vi "Test Copy from Pixmap ARGB.vi"(8 "error in (no error)":errorcluster, 11 "Test Case In":refnum<class "Image.lvclass">) -> (0 "error out":errorcluster, 3 "Test Case Out":refnum<class "Image.lvclass">)   [LabVIEW 2020, in "g_ar_toolkit.test.lvlib" / "Image.lvclass"]
uses:
  Image.lvclass
  C:/Program Files (x86)/National Instruments/LabVIEW 2020/vi.lib/Astemes/LUnit/Test Case.lvclass
  <vilib>/picture/picture.llb/imagedata.ctl
  <vilib>/Astemes/LUnit/Test Case.lvclass/Test Case.ctl
  2c93f62b-78d7-4b59-b27c-14bd701a5d71.vi
  26ba0610-68e5-456e-b31e-3dd4b1a41919.vi
  50a666bd-4679-4783-837b-c667b5268c61.vi
  5112621f-71fb-42da-a54b-011c251ba454.vi
  935961b4-3727-4f5b-bf0e-a61aebcf0dca.vi
  g_ar_toolkit.image/CreateEmptyImageARGB.vi
  g_ar_toolkit.image/CreateEmptyImageGreyscale.vi
  g_ar_toolkit.image/CopyPixmapToImageOuptutMaskARGB.vi
  g_ar_toolkit.image/CopyPixmapToImageFlattenMaskARGB.vi
  7f5bb767-9dbf-47d9-8f44-5f4901e96d00.vi
  e6d5ae8e-bd70-4c65-a769-b7cfb03e80c7.vi
  d454bffa-6717-48ab-b8d5-b1f03345aa55.vi
  g_ar_toolkit.image/CreateEmptyImageARGB.vi/3321fa97-f432-4e1e-8db9-a0df79aed21b.vi
  g_ar_toolkit.image/CreateEmptyImageGreyscale.vi/6598b9e0-8a08-46f5-91fd-ca1b87217137.vi
  g_ar_toolkit.image/CopyPixmapToImageOuptutMaskARGB.vi/80b1166a-8c06-443b-b271-eb6a715622f7.vi
  g_ar_toolkit.image/CopyPixmapToImageFlattenMaskARGB.vi/80b1166a-8c06-443b-b271-eb6a715622f7.vi
  <vilib>/Astemes/LUnit/Append Pass Result.vi
  <vilib>/Astemes/LUnit/Append Fail Result.vi
  <vilib>/Astemes/LUnit/Describe Comparison.vi
  <vilib>/Astemes/LUnit/Compare Variants.vi
  g_ar_toolkit.image/FixPixmap.vi
  <vilib>/Astemes/LUnit/Variant to string.vi
  g_ar_toolkit.image/Default8bitColourMap.vi
  g_ar_toolkit.image/ARGBColourToU32.vi
  <vilib>/Utility/error.llb/Error Cluster From Error Code.vi
  <vilib>/Utility/Data Type/Get Type Information.vi
  <vilib>/Utility/LVClass/Get LV Class Name.vi
  Image.lvclass/Image.ctl
  g_ar_toolkit.image/g_ar_toolkit.image.lvlib
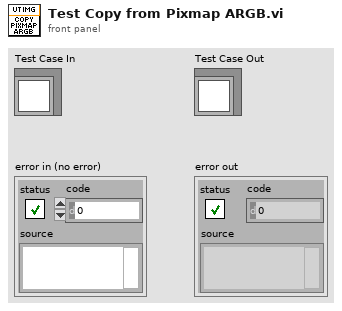
[diagram p1: front panel]
types:
  T1 = enum16{"8 Bit No Mask", "24 Bit No Mask", "32 Bit No Mask", "8 Bit Mask", "24 Bit Mask", "32 Bit Mask", "8 Pixels Wide Masked", "16 Pixels Wide Masked", "8 Bit No Colour Map"}
  T2 = typedef "imagedata.ctl" = cluster{"image type":i32, "image depth":i32, "image":u8[], "mask":u8[], "colors":u32[], "Rectangle":cluster{"left":i16, "top":i16, "right":i16, "bottom":i16}}
  T3 = cluster{"8 No Mask":T2, "8 Mask":T2, "24 No Mask":T2, "24 Mask":T2, "32 No Mask":T2, "32 Mask":T2, "24 Mask - 8 wide":T2, "24 Mask - 16 wide":T2, "8 Bit No Colour Map":T2}
  T4 = cluster{"left":i16, "top":i16, "right":i16, "bottom":i16}
  T5 = enum16{"8 Bit No Mask", "24 Bit No Mask", "32 Bit No Mask", "8 Bit Mask", "24 Bit Mask", "32 Bit Mask", "8 Pixels Wide Masked", "16 Pixels Wide Masked", "8 Bit No Colour Map"}[]
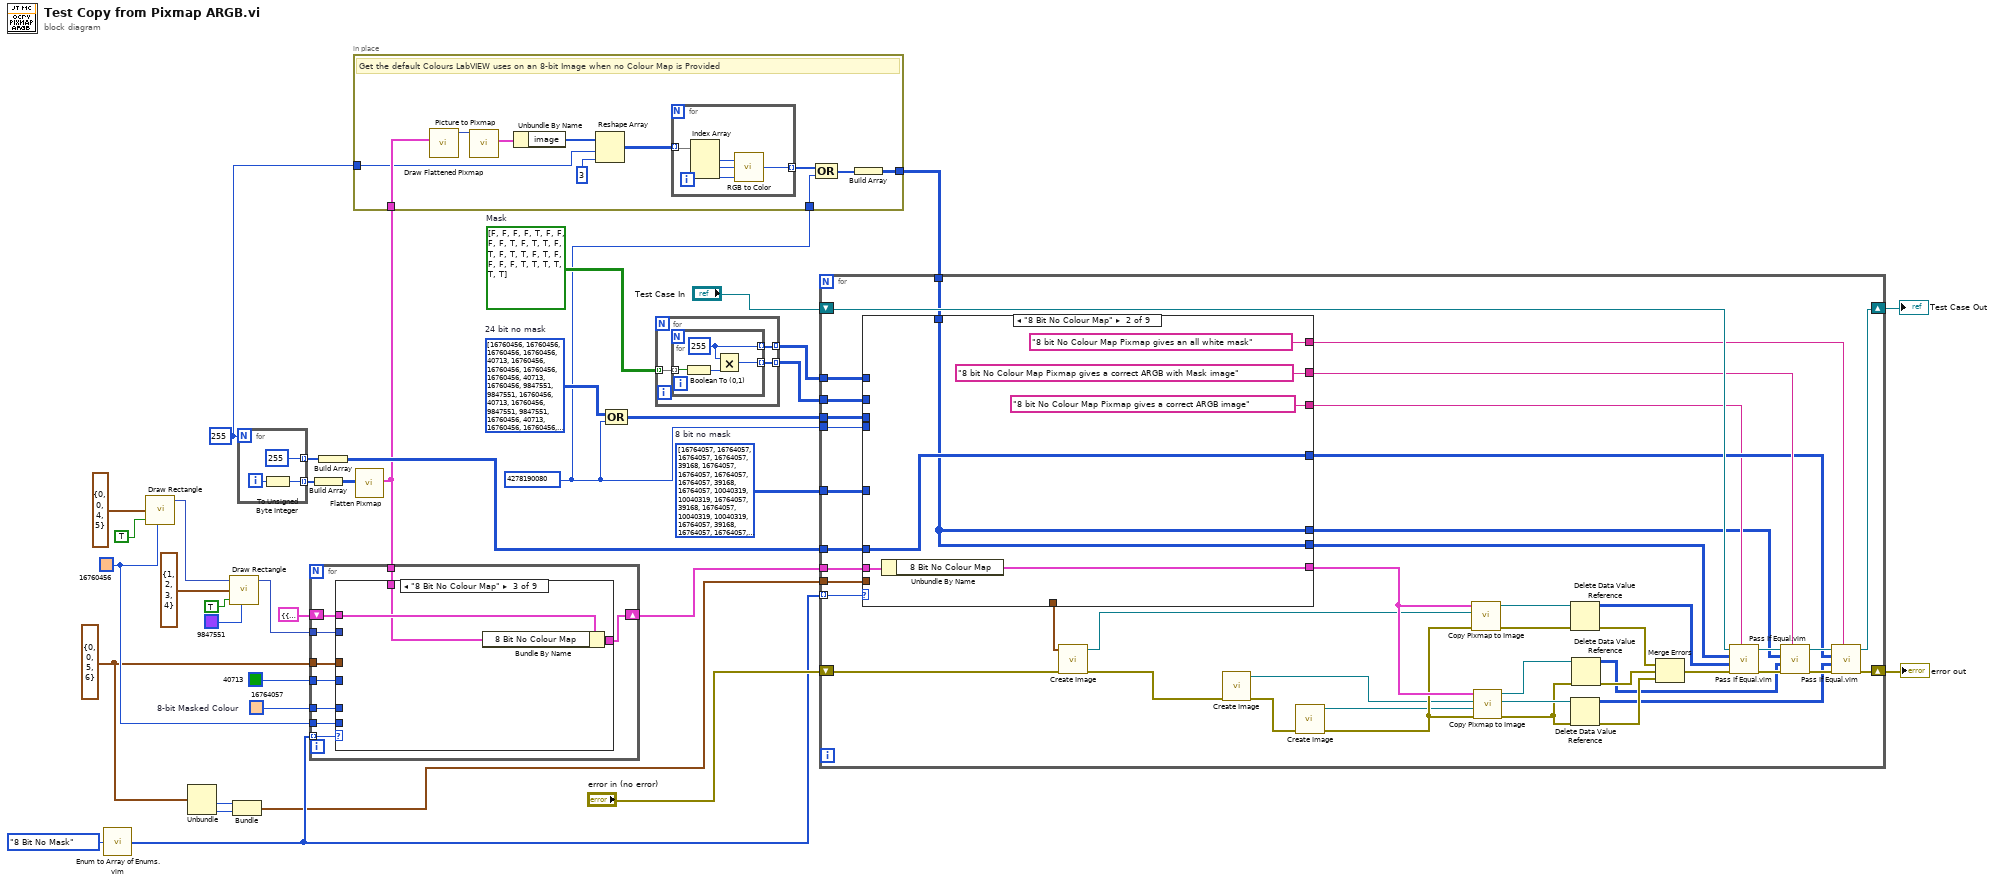
[diagram p0: block diagram]
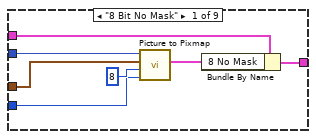
[diagram p2: hidden frame]
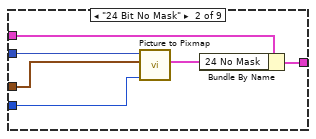
[diagram p3: hidden frame]
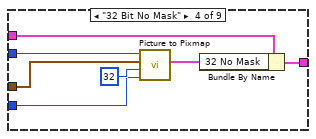
[diagram p4: hidden frame]
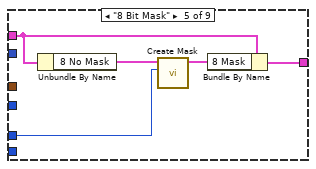
[diagram p5: hidden frame]
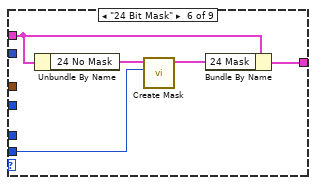
[diagram p6: hidden frame]
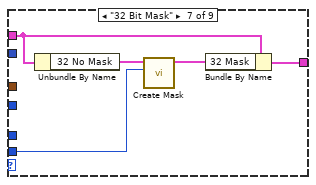
[diagram p7: hidden frame]
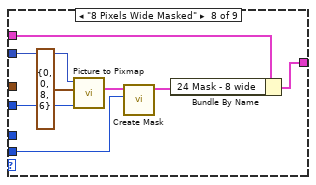
[diagram p8: hidden frame]
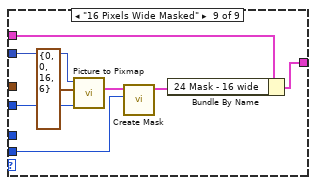
[diagram p9: hidden frame]
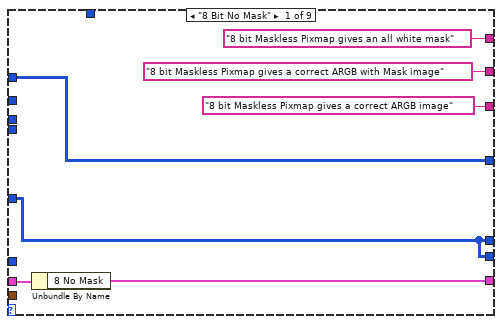
[diagram p10: hidden frame]
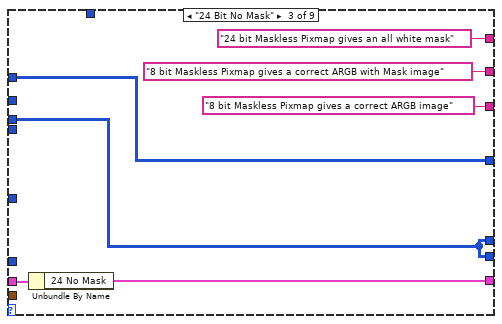
[diagram p11: hidden frame]
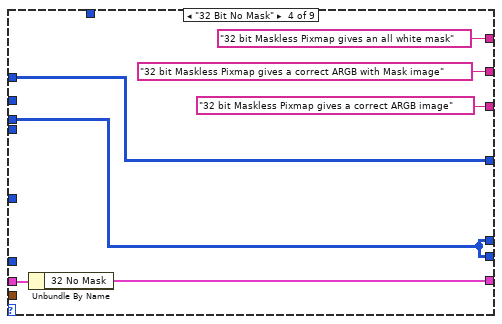
[diagram p12: hidden frame]
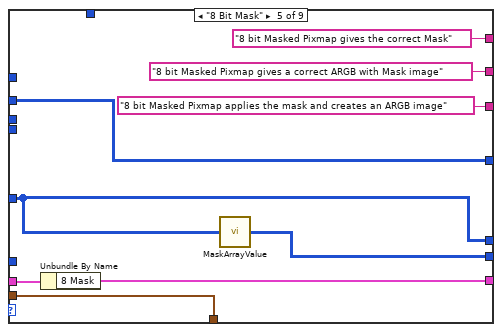
[diagram p13: hidden frame]
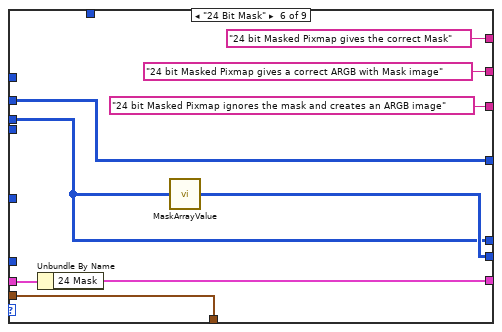
[diagram p14: hidden frame]
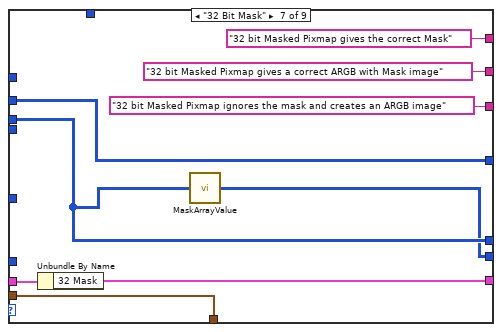
[diagram p15: hidden frame]
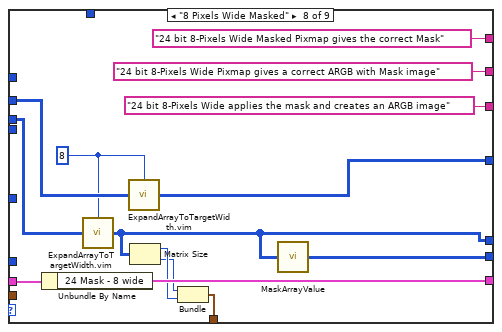
[diagram p16: hidden frame]
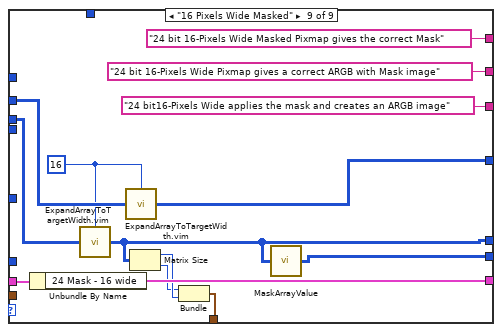
[diagram p17: hidden frame]
diagram:
  w1 = 255
  w9 = u32 16764057  # 8-bit Masked Colour
  w23 = bool[][] [[FALSE, FALSE, FALSE, FALSE, TRUE], [FALSE, FALSE, FALSE, FALSE, TRUE], [FALSE, TRUE, TRUE, FALSE, TRUE], [FALSE, TRUE, TRUE, FALSE, TRUE], [FALSE, FALSE, FALSE, FALSE, TRUE], [TRUE, TRUE, TRUE, TRUE, TRUE]]  # Mask
  w10 = u32[][] [[16764057, 16764057, 16764057, 16764057, 39168], [16764057, 16764057, 16764057, 16764057, 39168], [16764057, 10040319, 10040319, 16764057, 39168], [16764057, 10040319, 10040319, 16764057, 39168], [16764057, 16764057, 16764057, 16764057, 39168], [39168, 39168, 39168, 39168, 39168]]  # 8 bit no mask
  w2 = u32 4278190080
  w26 = u32[][] [[16760456, 16760456, 16760456, 16760456, 40713], [16760456, 16760456, 16760456, 16760456, 40713], [16760456, 9847551, 9847551, 16760456, 40713], [16760456, 9847551, 9847551, 16760456, 40713], [16760456, 16760456, 16760456, 16760456, 40713], [40713, 40713, 40713, 40713, 40713]]  # 24 bit no mask
  w14 = T4 {"left"=0, "top"=0, "right"=5, "bottom"=6} ("rect")
  w17 = u32 16760456 ("color(black)")
  n1 = call "Enum to Array of Enums.vim"("enum"=T1."8 Bit No Mask") -> ("array of enums"=w21:T5)
  n2 = call <vilib>:"Draw Rectangle.vi"("rect"=T4 {"left"=0, "top"=0, "right"=4, "bottom"=5}, "fill?(F)"=TRUE, "color(black)"=w17) -> ("new picture"=w36:picture)  [unwired: 6 in]
  n3 = Unbundle(w14) -> ("right"=w13:i16, "bottom"=w12:i16)  [unwired: 2 out]
  n4 = call <vilib>:"Draw Rectangle.vi"("picture"=w36, "rect"=T4 {"left"=1, "top"=2, "right"=3, "bottom"=4}, "fill?(F)"=TRUE, "color(black)"=u32 9847551) -> ("new picture"=w18:picture)  [unwired: 5 in]
  n5 = Bundle("right"=w13, "bottom"=w12) -> (w11:cluster{"right":i16, "bottom":i16})  [unwired: 1 in]
  n6 = for {
    N: w1 -> [_]
    tunnel: [w38] -> w8 mode=indexing
    tunnel: [u8 255 ("unsigned 8bit integer")] -> w6 mode=indexing
    i -> [w39]
    n7 = To Unsigned Byte Integer(number=w39) -> (unsigned 8bit integer=w38:u8)
  }
  n8 = Build Array(w8) -> (w7:u8[][])
  n9 = Build Array(w6) -> (w5:u8[][])
  n10 = call <vilib>:"Flatten Pixmap.vi"("8-bit pixmap"=w7) -> ("image data"=w4:T2)  [unwired: 10 in]
  n11 = for {
    tunnel: w21 -> [w46] mode=indexing
    shift-right: [w47] -> w19
    shift-left: T3 {"8 No Mask"={"image type"=0, "image depth"=0, "image"=[], "mask"=[], "colors"=[], "Rectangle"={"left"=0, "top"=0, "right"=0, "bottom"=0}}, "8 Mask"={"image type"=0, "image depth"=0, "image"=[], "mask"=[], "colors"=[], "Rectangle"={"left"=0, "top"=0, "right"=0, "bottom"=0}}, "24 No Mask"={"image type"=0, "image depth"=0, "image"=[], "mask"=[], "colors"=[], "Rectangle"={"left"=0, "top"=0, "right"=0, "bottom"=0}}, "24 Mask"={"image type"=0, "image depth"=0, "image"=[], "mask"=[], "colors"=[], "Rectangle"={"left"=0, "top"=0, "right"=0, "bottom"=0}}, "32 No Mask"={"image type"=0, "image depth"=0, "image"=[], "mask"=[], "colors"=[], "Rectangle"={"left"=0, "top"=0, "right"=0, "bottom"=0}}, "32 Mask"={"image type"=0, "image depth"=0, "image"=[], "mask"=[], "colors"=[], "Rectangle"={"left"=0, "top"=0, "right"=0, "bottom"=0}}, "24 Mask - 8 wide"={"image type"=0, "image depth"=0, "image"=[], "mask"=[], "colors"=[], "Rectangle"={"left"=0, "top"=0, "right"=0, "bottom"=0}}, "24 Mask - 16 wide"={"image type"=0, "image depth"=0, "image"=[], "mask"=[], "colors"=[], "Rectangle"={"left"=0, "top"=0, "right"=0, "bottom"=0}}, "8 Bit No Colour Map"={"image type"=0, "image depth"=0, "image"=[], "mask"=[], "colors"=[], "Rectangle"={"left"=0, "top"=0, "right"=0, "bottom"=0}}} ("output cluster") -> [w48]
    tunnel: w18 -> [w44]
    tunnel: w14 -> [w45]
    tunnel: u32 40713 ("Background Color") -> [w43]
    tunnel: w17 -> [w42]
    tunnel: w9 -> [w41]
    tunnel: w4 -> [w40]
    n12 = case shown="\"8 Bit No Colour Map\"" w46 {
      tunnel: w48 -> [w55 w61 w64 w71 w75 w80 w85 w94 w102]
      tunnel: [w54 w60 w63 w70 w76 w81 w86 w93 w101] -> w47
      tunnel: w45 -> [w52 w59 _ w68 _ _ _ _ _]
      tunnel: w44 -> [w51 w58 _ w67 _ _ _ w90 w98]
      tunnel: w43 -> [w49 w56 _ w65 _ _ _ w89 w97]
      tunnel: w42 -> [_ _ _ _ _ w77 w82 w87 w95]
      tunnel: w41 -> [_ _ _ _ w72 _ _ _ _]
      tunnel: w40 -> [_ _ w62 _ _ _ _ _ _]
      frame "8 Bit No Mask" {
        n13 = call <vilib>:"Picture to Pixmap.vi"("Background Color"=w49, "depth"=8, "rect"=w52, "picture"=w51) -> ("image data"=w50:T2)  [unwired: 6 in, 1 out]
        n14 = Bundle By Name(cluster=w55, "8 No Mask"=w50) -> (w54:T3)
      }
      frame "24 Bit No Mask" {
        n15 = call <vilib>:"Picture to Pixmap.vi"("Background Color"=w56, "rect"=w59, "picture"=w58) -> ("image data"=w57:T2)  [unwired: 7 in, 1 out]
        n16 = Bundle By Name(cluster=w61, "24 No Mask"=w57) -> (w60:T3)
      }
      frame "8 Bit No Colour Map" {
        n17 = Bundle By Name(cluster=w64, "8 Bit No Colour Map"=w62) -> (w63:T3)
      }
      frame "32 Bit No Mask" {
        n18 = call <vilib>:"Picture to Pixmap.vi"("Background Color"=w65, "depth"=32, "rect"=w68, "picture"=w67) -> ("image data"=w66:T2)  [unwired: 6 in, 1 out]
        n19 = Bundle By Name(cluster=w71, "32 No Mask"=w66) -> (w70:T3)
      }
      frame "8 Bit Mask" {
        n20 = Unbundle By Name(w75) -> ("8 No Mask"=w74:T2)
        n21 = call <vilib>:"Create Mask.vi"("Mask Color (Black)"=w72, "image data"=w74) -> ("image data"=w73:T2)  [unwired: 9 in]
        n22 = Bundle By Name(cluster=w75, "8 Mask"=w73) -> (w76:T3)
      }
      frame "24 Bit Mask" {
        n23 = Unbundle By Name(w80) -> ("24 No Mask"=w79:T2)
        n24 = call <vilib>:"Create Mask.vi"("Mask Color (Black)"=w77, "image data"=w79) -> ("image data"=w78:T2)  [unwired: 9 in]
        n25 = Bundle By Name(cluster=w80, "24 Mask"=w78) -> (w81:T3)
      }
      frame "32 Bit Mask" {
        n26 = Unbundle By Name(w85) -> ("32 No Mask"=w84:T2)
        n27 = call <vilib>:"Create Mask.vi"("Mask Color (Black)"=w82, "image data"=w84) -> ("image data"=w83:T2)  [unwired: 9 in]
        n28 = Bundle By Name(cluster=w85, "32 Mask"=w83) -> (w86:T3)
      }
      frame "8 Pixels Wide Masked" {
        n29 = call <vilib>:"Picture to Pixmap.vi"("Background Color"=w89, "rect"=T4 {"left"=0, "top"=0, "right"=8, "bottom"=6}, "picture"=w90) -> ("image data"=w92:T2)  [unwired: 7 in, 1 out]
        n30 = call <vilib>:"Create Mask.vi"("Mask Color (Black)"=w87, "image data"=w92) -> ("image data"=w91:T2)  [unwired: 9 in]
        n31 = Bundle By Name(cluster=w94, "24 Mask - 8 wide"=w91) -> (w93:T3)
      }
      frame "16 Pixels Wide Masked" {
        n32 = call <vilib>:"Picture to Pixmap.vi"("Background Color"=w97, "rect"=T4 {"left"=0, "top"=0, "right"=16, "bottom"=6}, "picture"=w98) -> ("image data"=w100:T2)  [unwired: 7 in, 1 out]
        n33 = call <vilib>:"Create Mask.vi"("Mask Color (Black)"=w95, "image data"=w100) -> ("image data"=w99:T2)  [unwired: 9 in]
        n34 = Bundle By Name(cluster=w102, "24 Mask - 16 wide"=w99) -> (w101:T3)
      }
    }
  }
  n35 = in-place {
    in-place-border: w4 -> [w113]
    in-place-border: [w109] -> w3
    in-place-border: w2 -> [w106]
    in-place-border: w1 -> [w103]
    # "Get the default Colours LabVIEW uses on an 8-bit Image when no Colour Map is Provided"
    n36 = call <vilib>:"Draw Flattened Pixmap.vi"("image data"=w113) -> ("new picture"=w112:picture)  [unwired: 8 in]
    n37 = call <vilib>:"Picture to Pixmap.vi"("picture"=w112) -> ("image data"=w111:T2)  [unwired: 9 in, 1 out]
    n38 = Unbundle By Name(w111) -> ("image"=w110:u8[])
    n39 = Reshape Array(w110, w103, 3 ("dimension size")) -> (w105:u8[][])
    n40 = for {
      tunnel: w105 -> [w118] mode=indexing
      tunnel: [w114] -> w108 mode=indexing
      n41 = Index Array(array=w118) -> (element #1=w116:u8, element #2=w117:u8, element #3=w115:u8)  [unwired: 3 in]
      n42 = call <vilib>:"RGB to Color.vi"("B"=w115, "G"=w117, "R"=w116) -> ("Color"=w114:u32)
    }
    n43 = Compound Arithmetic op=OR(w108, w106) -> (w107:u32[])
    n44 = Build Array(w107) -> (w109:u32[][])
  }
  n45 = Compound Arithmetic op=OR(w26, w2) -> (w25:u32[][])
  n46 = for "Masks" {
    tunnel: w23 -> [w120] mode=indexing
    tunnel: [w121] -> w24 mode=indexing
    tunnel: [w119] -> w22 mode=indexing
    n47 = for {
      tunnel: [w124] -> w121 mode=indexing
      tunnel: w120 -> [w125] mode=indexing
      tunnel: [w123] -> w119 mode=indexing
      w124 = u8 255 ("unsigned 8bit integer")
      n48 = Boolean To (0,1)(Boolean=w125) -> (0, 1=w122:i16)
      n49 = Multiply(x=w124, y=w122) -> (x*y=w123:u8)
    }
  }
  n50 = for {
    tunnel: w19 -> [w169]
    tunnel: w21 -> [w163] mode=indexing
    shift-right: [w154] -> w27
    shift-left: "error in (no error)" -> [w146]
    shift-right: [w153] -> w30
    shift-left: "Test Case In" -> [w162]
    tunnel: w25 -> [w147]
    tunnel: w10 -> [w150]
    tunnel: w24 -> [w143]
    tunnel: w22 -> [w142]
    tunnel: w11 -> [w137]
    tunnel: w2 -> [w130]
    tunnel: w5 -> [w127]
    tunnel: w3 -> [w126]
    n51 = case shown="\"8 Bit No Colour Map\"" w163 {
      tunnel: w169 -> [w176 w183 w190 w197 w206 w215 w224 w238 w252]
      tunnel: [w175 w182 w189 w196 w205 w214 w223 w237 w251] -> w168
      tunnel: ["8 bit Maskless Pixmap gives an all white mask" ("Description") "8 bit No Colour Map Pixmap gives an all white mask" ("Description") "24 bit Maskless Pixmap gives an all white mask" ("Description") "32 bit Maskless Pixmap gives an all white mask" ("Description") "8 bit Masked Pixmap gives the correct Mask" ("Description") "24 bit Masked Pixmap gives the correct Mask" ("Description") "32 bit Masked Pixmap gives the correct Mask" ("Description") "24 bit 8-Pixels Wide Masked Pixmap gives the correct Mask" ("Description") "24 bit 16-Pixels Wide Masked Pixmap gives the correct Mask" ("Description")] -> w152
      tunnel: ["8 bit Maskless Pixmap gives a correct ARGB with Mask image" ("Description") "8 bit No Colour Map Pixmap gives a correct ARGB with Mask image" ("Description") "8 bit Maskless Pixmap gives a correct ARGB with Mask image" ("Description") "32 bit Maskless Pixmap gives a correct ARGB with Mask image" ("Description") "8 bit Masked Pixmap gives a correct ARGB with Mask image" ("Description") "24 bit Masked Pixmap gives a correct ARGB with Mask image" ("Description") "32 bit Masked Pixmap gives a correct ARGB with Mask image" ("Description") "24 bit 8-Pixels Wide Pixmap gives a correct ARGB with Mask image" ("Description") "24 bit 16-Pixels Wide Pixmap gives a correct ARGB with Mask image" ("Description")] -> w151
      tunnel: [w172 w177 w184 w191 w199 w208 w217 w225 w239] -> w129
      tunnel: w150 -> [w172 _ _ _ w198 _ _ _ _]
      tunnel: [w172 w177 w184 w191 w198 w207 w218 w226 w240] -> w131
      tunnel: [w170 w178 w185 w192 w201 w210 w219 w231 w245] -> w149
      tunnel: ["8 bit Maskless Pixmap gives a correct ARGB image" ("Description") "8 bit No Colour Map Pixmap gives a correct ARGB image" ("Description") "8 bit Maskless Pixmap gives a correct ARGB image" ("Description") "32 bit Maskless Pixmap gives a correct ARGB image" ("Description") "8 bit Masked Pixmap applies the mask and creates an ARGB image" ("Description") "24 bit Masked Pixmap ignores the mask and creates an ARGB image" ("Description") "32 bit Masked Pixmap ignores the mask and creates an ARGB image" ("Description") "24 bit 8-Pixels Wide applies the mask and creates an ARGB image" ("Description") "24 bit16-Pixels Wide applies the mask and creates an ARGB image" ("Description")] -> w148
      tunnel: w147 -> [_ _ w184 w191 _ w207 w218 w233 w247]
      tunnel: w143 -> [w170 _ w185 w192 _ _ _ _ _]
      tunnel: w142 -> [_ _ _ _ w201 w210 w219 w232 w246]
      tunnel: [_ _ _ _ w200 w209 w216 w227 w241] -> w138
      tunnel: w137 -> [_ _ _ _ w200 w209 w216 _ _]
      tunnel: w130 -> [_ _ _ _ _ _ _ _ _]
      tunnel: w127 -> [_ w178 _ _ _ _ _ _ _]
      tunnel: w126 -> [_ w177 _ _ _ _ _ _ _]
      frame "8 Bit No Mask" {
        n52 = Unbundle By Name(w176) -> ("8 No Mask"=w175:T2)
      }
      frame "8 Bit No Colour Map" {
        n53 = Unbundle By Name(w183) -> ("8 Bit No Colour Map"=w182:T2)
      }
      frame "24 Bit No Mask" {
        n54 = Unbundle By Name(w190) -> ("24 No Mask"=w189:T2)
      }
      frame "32 Bit No Mask" {
        n55 = Unbundle By Name(w197) -> ("32 No Mask"=w196:T2)
      }
      frame "8 Bit Mask" {
        n56 = Unbundle By Name(w206) -> ("8 Mask"=w205:T2)
        n57 = call "MaskArrayValue.vi"("Array In"=w198) -> ("Array out"=w199:u32[][])
      }
      frame "24 Bit Mask" {
        n58 = Unbundle By Name(w215) -> ("24 Mask"=w214:T2)
        n59 = call "MaskArrayValue.vi"("Array In"=w207) -> ("Array out"=w208:u32[][])
      }
      frame "32 Bit Mask" {
        n60 = Unbundle By Name(w224) -> ("32 Mask"=w223:T2)
        n61 = call "MaskArrayValue.vi"("Array In"=w218) -> ("Array out"=w217:u32[][])
      }
      frame "8 Pixels Wide Masked" {
        w230 = 8 ("Target Width")
        n62 = Unbundle By Name(w238) -> ("24 Mask - 8 wide"=w237:T2)
        n63 = call "ExpandArrayToTargetWidth.vim"("Array in"=w233, "Target Width"=w230) -> ("Array out"=w226:u32[][])
        n64 = call "ExpandArrayToTargetWidth.vim"("Array in"=w232, "Target Width"=w230) -> ("Array out"=w231:u8[][])
        n65 = Matrix Size(0:w226) -> (1:w229:i32, 2:w228:i32)
        n66 = Bundle("matrix"=w228, "number of columns"=w229) -> (w227:cluster{"matrix":i32, "number of columns":i32})  [unwired: 1 in]
        n67 = call "MaskArrayValue.vi"("Array In"=w226) -> ("Array out"=w225:u32[][])
      }
      frame "16 Pixels Wide Masked" {
        w244 = 16 ("Target Width")
        n68 = Unbundle By Name(w252) -> ("24 Mask - 16 wide"=w251:T2)
        n69 = call "ExpandArrayToTargetWidth.vim"("Array in"=w247, "Target Width"=w244) -> ("Array out"=w240:u32[][])
        n70 = call "ExpandArrayToTargetWidth.vim"("Array in"=w246, "Target Width"=w244) -> ("Array out"=w245:u8[][])
        n71 = Matrix Size(0:w240) -> (1:w243:i32, 2:w242:i32)
        n72 = Bundle("matrix"=w242, "number of columns"=w243) -> (w241:cluster{"matrix":i32, "number of columns":i32})  [unwired: 1 in]
        n73 = call "MaskArrayValue.vi"("Array In"=w240) -> ("Array out"=w239:u32[][])
      }
    }
    n74 = call-poly "Create Image.vi"("error in (no error)"=w146, "Preallocated Image Size (Default: 0,0)"=w138) -> ("error out"=w145:errorcluster, "New ARGB Image"=w144:refnum<data-value>)  [unwired: 8 in]
    n75 = call-poly "Create Image.vi"("error in (no error)"=w145) -> ("error out"=w141:errorcluster, "New ARGB Image"=w139:refnum<data-value>)  [unwired: 9 in]
    n76 = call-poly "Create Image.vi"("error in (no error)"=w141) -> ("error out"=w167:errorcluster, "New Greyscale Image"=w140:refnum<data-value>)  [unwired: 9 in]
    n77 = call-poly "Copy Pixmap to Image.vi"("error in (no error)"=w167, "ARGB Image Destination"=w144, "Pixmap Image Data"=w168) -> ("error out"=w133:errorcluster, "ARGB Image Destination (duplicate)"=w132:refnum<data-value>)  [unwired: 7 in]
    n78 = call-poly "Copy Pixmap to Image.vi"("error in (no error)"=w167, "Greyscale Image Mask"=w140, "ARGB Image Destination"=w139, "Pixmap Image Data"=w168) -> ("error out"=w135:errorcluster, "Greyscale Image Mask (duplicate)"=w136:refnum<data-value>, "ARGB Image Destination (duplicate)"=w134:refnum<data-value>)  [unwired: 5 in]
    n79 = Delete Data Value Reference(data value reference=w132, error in=w133) -> (data value=w128:u32[][], error out=w166:errorcluster)
    n80 = Delete Data Value Reference(data value reference=w136, error in=w135) -> (data value=w156:u8[][], error out=w164:errorcluster)
    n81 = Delete Data Value Reference(data value reference=w134, error in=w135) -> (data value=w157:u32[][], error out=w165:errorcluster)
    n82 = Merge Errors(w166, w165, w164) -> (w155:errorcluster)
    n83 = call "Pass If Equal.vim"("Description"=w148, "error in (no error)"=w155, "Actual"=w128, "Expected"=w129, "LUnit Test Case In"=w162) -> ("error out"=w159:errorcluster, "LUnit Test Case Out"=w161:refnum<class "Image.lvclass">)  [unwired: 5 in]
    n84 = call "Pass If Equal.vim"("Description"=w151, "error in (no error)"=w159, "Actual"=w157, "Expected"=w131, "LUnit Test Case In"=w161) -> ("error out"=w158:errorcluster, "LUnit Test Case Out"=w160:refnum<class "Image.lvclass">)  [unwired: 5 in]
    n85 = call "Pass If Equal.vim"("Description"=w152, "error in (no error)"=w158, "Actual"=w156, "Expected"=w149, "LUnit Test Case In"=w160) -> ("error out"=w154:errorcluster, "LUnit Test Case Out"=w153:refnum<class "Image.lvclass">)  [unwired: 5 in]
  }
  "error out" <- w27
  "Test Case Out" <- w30
